vi "fixfilename.vi"(9 "file extension":string="csv", 11 "Path":path) -> (2 "fixed path (string)":string, 3 "fixed path":path)   [LabVIEW 2012]
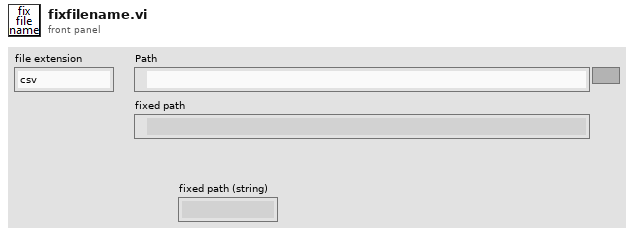
[diagram p1: front panel]
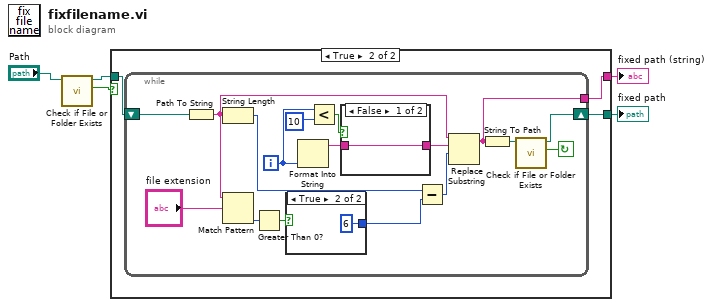
[diagram p0: block diagram]
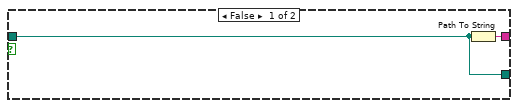
[diagram p2: hidden frame]
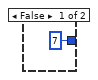
[diagram p3: hidden frame]
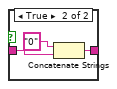
[diagram p4: hidden frame]
diagram:
  n1 = call <vilib>:"Check if File or Folder Exists.vi"("path"="Path") -> ("file or folder exists?"=w5:bool, "dup path"=w1:path)  [unwired: 8 in, 1 out]
  n2 = case shown="True" w5 {
    tunnel: [w7 w10] -> w4
    tunnel: w1 -> [w7 w9]
    tunnel: [w6 w8] -> w3
    frame False {
      n3 = Path To String(path=w7) -> (string=w6:string)
    }
    frame True {
      n4 = while {
        shift-right: [w11] -> w10
        shift-left: w9 -> [w19]
        tunnel: [w18] -> w8
        i -> [w26]
        stop <- w21 continue-if-true
        n5 = Path To String(path=w19) -> (string=w15:string)
        n6 = String Length(string=w15) -> (length=w17:i32)
        n7 = Match Pattern(string=w15, regular expression="file extension") -> (offset past match=w16:i32)  [unwired: 1 in, 3 out]
        n8 = Greater Than 0?(x=w16) -> (x > 0?=w14:bool)
        n9 = case shown="True" w14 {
          tunnel: [7 ("y") 6 ("y")] -> w13
          frame False {
          }
          frame True {
          }
        }
        n10 = Format Into String(w26) -> (resulting string=w23:string)  [unwired: 3 in, 1 out]
        n11 = Less?(x=w26, y=10) -> (x < y?=w24:bool)
        n12 = case shown="False" w24 {
          tunnel: w23 -> [w30 w32]
          tunnel: [w30 w31] -> w22
          frame False {
          }
          frame True {
            n13 = Concatenate Strings("0" ("string"), w32) -> (w31:string)
          }
        }
        n14 = Subtract(x=w17, y=w13) -> (x-y=w27:i32)
        n15 = Replace Substring(3:w27, 4:w22, 5:w15) -> (1:w18:string)  [unwired: 1 in, 1 out]
        n16 = String To Path(string=w18) -> (path=w20:path)
        n17 = call <vilib>:"Check if File or Folder Exists.vi"("path"=w20) -> ("file or folder exists?"=w21:bool, "dup path"=w11:path)  [unwired: 8 in, 1 out]
      }
    }
  }
  "fixed path" <- w4
  "fixed path (string)" <- w3
